vi "Pre Launch Init.vi"(11 "Simulated Entry Console Actor in":refnum<class "Simulated Entry Console Actor.lvclass">) -> (0 "error out":errorcluster, 3 "Simulated Entry Console Actor out":refnum<class "Simulated Entry Console Actor.lvclass">)   [LabVIEW 2019, in "Simulated Entry Console Actor.lvlib" / "Simulated Entry Console Actor.lvclass"]
doc: "(<B>Filename</B>: Actor Framework.lvlib:Actor.lvclass:Pre Launch Init.vi)\n\nDefines behavior that occurs after the Launch Nested Actor method is invoked but before the actor's Actor Core method begins running.\n\nBy default, this method does nothing. A descendant class may override it to define behavior."
uses:
  Simulated Entry Console Actor.lvclass
  Simulated Entry Console Actor.lvclass/Simulated Entry Console Actor.ctl
  Abstract Entry Console Actor/Abstract Entry Console Actor/Entry Console Actor.lvclass
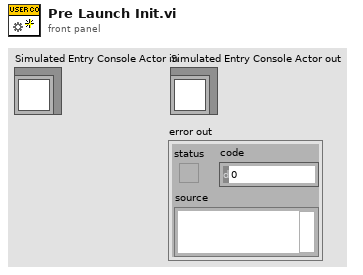
[diagram p1: front panel]
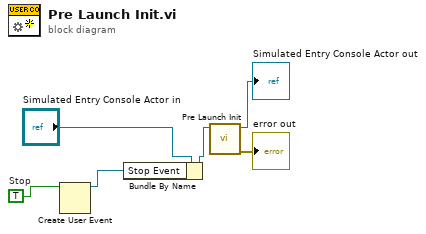
[diagram p0: block diagram]
diagram:
  w4 = TRUE  # Stop
  n1 = Create User Event(user event datatype=w4) -> (user event=w1:refnum<user-event>)  [unwired: 1 in, 1 out]
  n2 = Bundle By Name(cluster="Simulated Entry Console Actor in", "Stop Event"=w1) -> (w2:refnum<class "Simulated Entry Console Actor.lvclass">)
  n3 = call-parent "Pre Launch Init.vi"("Actor in"=w2) -> ("error out"=→"error out":errorcluster, "Actor out"=→"Simulated Entry Console Actor out":refnum<class "Simulated Entry Console Actor.lvclass">)  [unwired: 9 in]
